vi "string shorten.vi"(9 "# of characters in the beginning":i32=4, 10 "# of characters in the end":i32=12, 11 "input":string="Cell9_SS_2017.009.txt") -> (3 "shortened":string="Cell9_SS,,.009.txt")   [LabVIEW 2020]
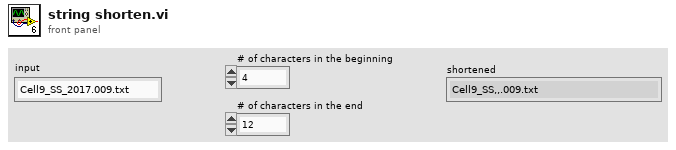
[diagram p1: front panel]
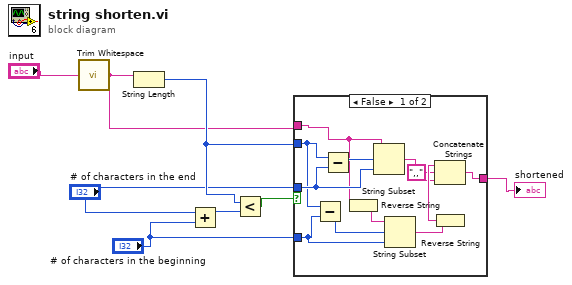
[diagram p0: block diagram]
diagram:
  n1 = call <vilib>:"Trim Whitespace.vi"("string"="input") -> ("trimmed string"=w3:string)  [unwired: 1 in]
  n2 = String Length(string=w3) -> (length=w6:i32)
  n3 = Add(x="# of characters in the end", y="# of characters in the beginning") -> (x+y=w8:i32)
  n4 = Less?(x=w6, y=w8) -> (x < y?=w7:bool)
  n5 = case shown="False" w7 {
    tunnel: [w18 w21] -> w2
    tunnel: w3 -> [w16 w21]
    tunnel: w6 -> [w15 _]
    tunnel: "# of characters in the end" -> [w20 _]
    tunnel: "# of characters in the beginning" -> [w14 _]
    frame False {
      n6 = Subtract(x=w15, y=w14) -> (x-y=w13:i32)
      n7 = Subtract(x=w15, y=w20) -> (x-y=w19:i32)
      n8 = Reverse String(1:w16) -> (0:w17:string)
      n9 = String Subset(string=w16, offset (0)=w19, length (rest)=w20) -> (substring=w10:string)
      n10 = String Subset(string=w17, offset (0)=w13, length (rest)=w14) -> (substring=w12:string)
      n11 = Reverse String(1:w12) -> (0:w11:string)
      n12 = Concatenate Strings(w11, ",," ("string"), w10) -> (w18:string)
    }
    frame True {
    }
  }
  "shortened" <- w2
